vi "FileManagement.vi"(1 "File Name":string, 2 "Target File Path":path, 3 "ezAFM Default Path":path=path "D:/ezAFM/Scanned Images") -> ()   [LabVIEW 2015]
panel:
  out "error out":errorcluster
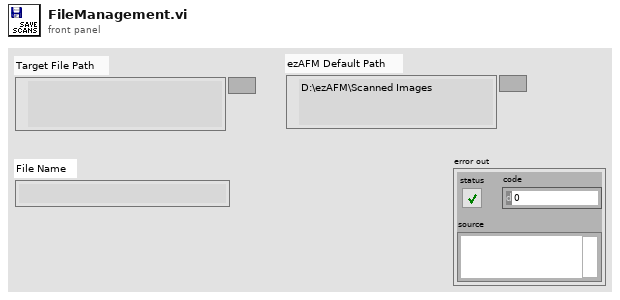
[diagram p1: front panel]
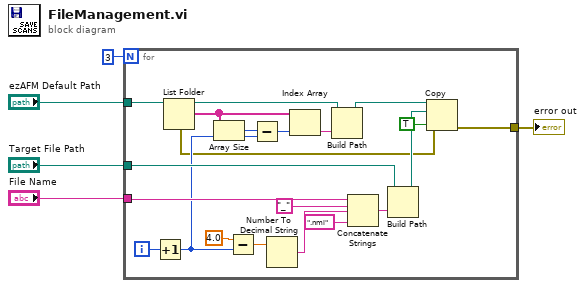
[diagram p0: block diagram]
diagram:
  n1 = for {
    N: 3 -> [_]
    tunnel: "ezAFM Default Path" -> [w21]
    tunnel: "Target File Path" -> [w20]
    tunnel: "File Name" -> [w17]
    tunnel: [w7] -> w1
    i -> [w19]
    n2 = Increment(x=w19) -> (x+1=w9:i32)
    n3 = List Folder(path=w21) -> (path out=w25:path, filenames=w8:string[], error out=w6:errorcluster)  [unwired: 3 in, 1 out]
    n4 = Array Size(array=w8) -> (size(s)=w14:i32)
    n5 = Subtract(x=4.0, y=w9) -> (x-y=w10:dbl)
    n6 = Subtract(x=w14, y=w9) -> (x-y=w13:i32)
    n7 = Number To Decimal String(number=w10) -> (decimal integer string=w15:string)  [unwired: 1 in]
    n8 = Index Array(array=w8, index=w13) -> (element=w26:string)
    n9 = Build Path(base path=w25, name or relative path=w26) -> (appended path=w24:path)
    n10 = Concatenate Strings(w17, "_" ("string"), w15, ".nmi" ("string")) -> (w16:string)
    n11 = Build Path(base path=w20, name or relative path=w16) -> (appended path=w23:path)
    n12 = Copy(8:w6, 9:TRUE ("overwrite (F)"), 10:w23, 11:w24) -> (0:w7:errorcluster)  [unwired: 1 in, 2 out]
  }
  "error out" <- w1
